vi "Close.vi"(8 "error in (no error)":errorcluster, 11 "PLBB in":refnum<class "PL BlackBox Modbus Client.lvclass">) -> (0 "error out":errorcluster)   [LabVIEW 2015, in "PL BlackBox Modbus Client.lvclass"]
doc: "Closes connection to device."
uses:
  PL BlackBox Modbus Client.lvclass
  <vilib>/plasmapper/PL Modbus Client/PL Modbus Client.lvclass
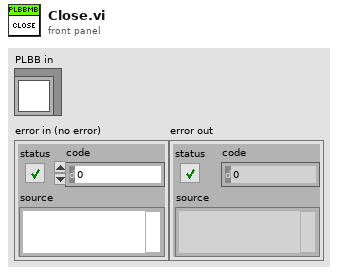
[diagram p1: front panel]
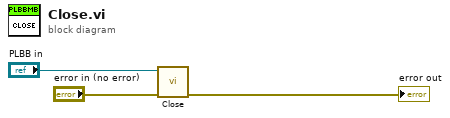
[diagram p0: block diagram]
diagram:
  n1 = call-parent "Close.vi"("error in (no error)"="error in (no error)", "MODBUS in"="PLBB in") -> ("error out"=→"error out":errorcluster)  [unwired: 9 in]
